vi "WheelShooter Shoot.vi"(1 "cluster in":T9, 2 "Range":dbl) -> (0 "error out":errorcluster)   [LabVIEW 2015]
doc: "Spins up the firing motors and then shoots over one second."
uses:
  <vilib>/Rock Robotics/WPI/MotorControl/WPI_MotorControlDeviceRef.ctl
  <vilib>/Rock Robotics/WPI/MotorControl/WPI_MotorControlType.ctl
  <vilib>/Rock Robotics/SystemInterfaces/DIO/FPGA_DIOPWMChannel.ctl
  <vilib>/Rock Robotics/WPI/PWM/WPI_PWMDeadband.ctl
  <vilib>/Rock Robotics/WPI/CAN/Jaguar/SubVIs/WPI_CANJaguar_ControlMode.ctl
  <vilib>/Rock Robotics/WPI/CAN/TalonSRX/WPI_CANTalonSRX_APIControlMode.ctl
  <vilib>/Rock Robotics/WPI/PWM/Servo/WPI_ServoDeviceRef.ctl
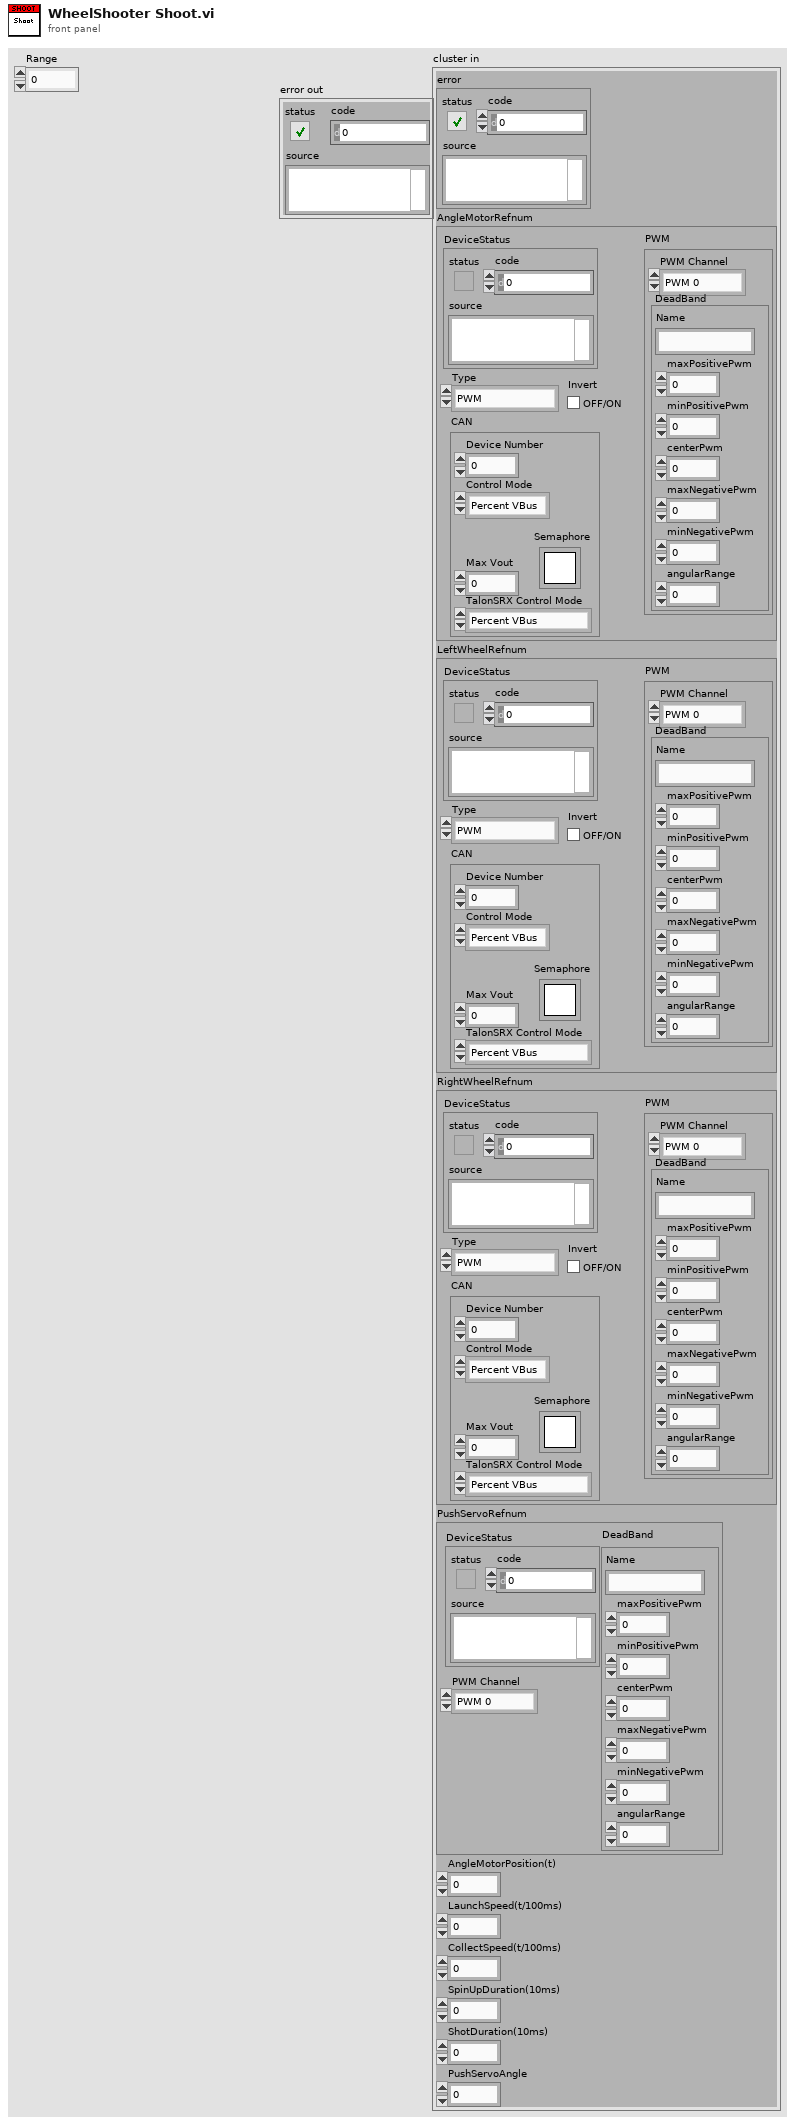
[diagram p1: front panel]
types:
  T1 = typedef "WPI_MotorControlDeviceRef.ctl" = cluster{"DeviceStatus":errorcluster, "Type":T2, "PWM":cluster{"PWM Channel":T3, "DeadBand":T4}, "CAN":cluster{"Device Number":u8, "Control Mode":T5, "Semaphore":T6, "Max Vout":dbl, "TalonSRX Control Mode":T7}, "Invert":bool}
  T2 = typedef "WPI_MotorControlType.ctl" = enum16{"PWM", "CAN", "CANTalonSRX"}
  T3 = typedef "FPGA_DIOPWMChannel.ctl" = enum8{"PWM 0", "PWM 1", "PWM 2", "PWM 3", "PWM 4", "PWM 5", "PWM 6", "PWM 7", "PWM 8", "PWM 9", "PWM MXP 0", "PWM MXP 1", "PWM MXP 2", "PWM MXP 3", "PWM MXP 4", "PWM MXP 5", "PWM MXP 6", "PWM MXP 7", "PWM MXP 8", "PWM MXP 9", "Invalid"}
  T4 = typedef "WPI_PWMDeadband.ctl" = cluster{"Name":string, "maxPositivePwm":i32, "minPositivePwm":i32, "centerPwm":i32, "maxNegativePwm":i32, "minNegativePwm":i32, "angularRange":u16}
  T5 = typedef "WPI_CANJaguar_ControlMode.ctl" = enum8{"Percent VBus", "Current", "Speed", "Position", "Voltage"}
  T6 = typedef "Semaphore RefNum" = refnum<k1>
  T7 = typedef "WPI_CANTalonSRX_APIControlMode.ctl" = enum8{"Percent VBus", "Speed", "Position", "Slave", "Unchanged / Invalid", "Voltage Compensation", "Current", "Motion Profile"}
  T8 = typedef "WPI_ServoDeviceRef.ctl" = cluster{"DeviceStatus":errorcluster, "PWM Channel":T3, "DeadBand":T4}
  T9 = cluster{"error":errorcluster, "AngleMotorRefnum":T1, "LeftWheelRefnum":T1, "RightWheelRefnum":T1, "PushServoRefnum":T8, "AngleMotorPosition(t)":dbl, "LaunchSpeed(t/100ms)":dbl, "CollectSpeed(t/100ms)":dbl, "SpinUpDuration(10ms)":i32, "ShotDuration(10ms)":i32, "PushServoAngle":i32}
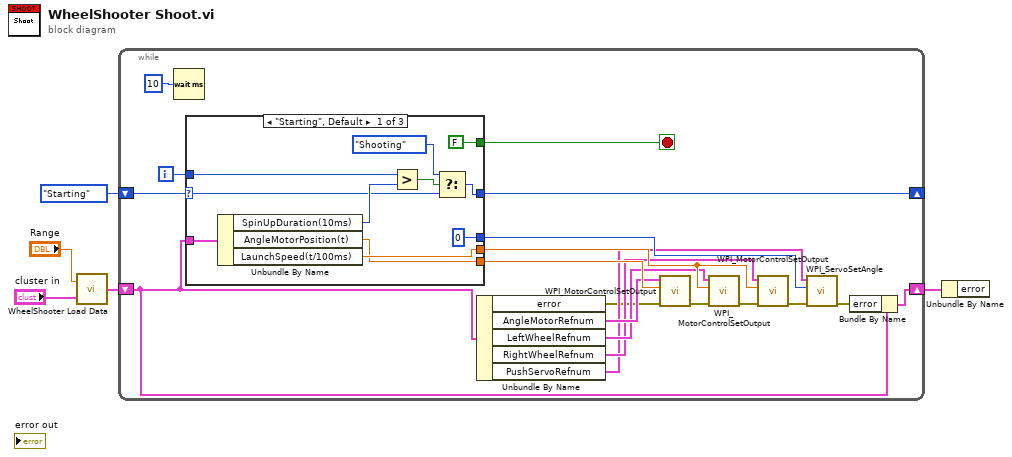
[diagram p0: block diagram]
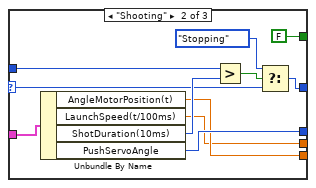
[diagram p2: hidden frame]
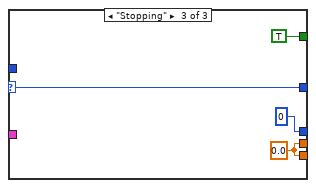
[diagram p3: hidden frame]
diagram:
  n1 = call "WheelShooter Load Data.vi"("cluster in"="cluster in", "Range"="Range") -> ("cluster out"=w3:T9)
  n2 = while {
    shift-right: [w20] -> _
    shift-left: enum16{"Starting", "Shooting", "Stopping"}."Starting" -> [w24]
    shift-right: [w13] -> w2
    shift-left: w3 -> [w12]
    i -> [w21]
    stop <- w6 stop-if-true
    n3 = Wait (ms)(milliseconds to wait=u32 10) -> ()  [unwired: 1 out]
    n4 = case shown="\"Starting\", Default" w24 {
      selector: w24 -> [w31 w43 w49]
      tunnel: [0 ("Angle") w40 0 ("Angle")] -> w23
      tunnel: w21 -> [w35 w44 _]
      tunnel: w12 -> [w33 w46 _]
      tunnel: [w29 w42 w49] -> w20
      tunnel: [w28 w37 w48] -> w19
      tunnel: [w27 w38 w48] -> w18
      tunnel: [FALSE FALSE TRUE] -> w6
      frame "Starting", Default {
        n5 = Unbundle By Name(w33) -> ("SpinUpDuration(10ms)"=w32:i32, "AngleMotorPosition(t)"=w27:dbl, "LaunchSpeed(t/100ms)"=w28:dbl)
        n6 = Greater?(x=w35, y=w32) -> (0:w30:bool)
        n7 = Select(t=enum16{"Starting", "Shooting", "Stopping"}."Shooting", s=w30, f=w31) -> (s? t:f=w29:enum16{"Starting", "Shooting", "Stopping"})
      }
      frame "Shooting" {
        n8 = Unbundle By Name(w46) -> ("AngleMotorPosition(t)"=w38:dbl, "LaunchSpeed(t/100ms)"=w37:dbl, "ShotDuration(10ms)"=w45:i32, "PushServoAngle"=w40:i32)
        n9 = Greater?(x=w44, y=w45) -> (0:w39:bool)
        n10 = Select(t=enum16{"Starting", "Shooting", "Stopping"}."Stopping", s=w39, f=w43) -> (s? t:f=w42:enum16{"Starting", "Shooting", "Stopping"})
      }
      frame "Stopping" {
        w48 = 0.0 ("AngleMotorT")
      }
    }
    n11 = Unbundle By Name(w12) -> ("error"=w7:errorcluster, "AngleMotorRefnum"=w17:T1, "LeftWheelRefnum"=w16:T1, "RightWheelRefnum"=w15:T1, "PushServoRefnum"=w14:T8)
    n12 = call <vilib>:"WPI_MotorControlSetOutput.vi"("error in (no error)"=w7, "Output"=w18, "MotorControlDevRef"=w17) -> ("error out"=w8:errorcluster)  [unwired: 6 in, 2 out]
    n13 = call <vilib>:"WPI_MotorControlSetOutput.vi"("error in (no error)"=w8, "Output"=w19, "MotorControlDevRef"=w16) -> ("error out"=w9:errorcluster)  [unwired: 6 in, 2 out]
    n14 = call <vilib>:"WPI_MotorControlSetOutput.vi"("error in (no error)"=w9, "Output"=w19, "MotorControlDevRef"=w15) -> ("error out"=w10:errorcluster)  [unwired: 6 in, 2 out]
    n15 = call <vilib>:"WPI_ServoSetAngle.vi"("error in (no error)"=w10, "Angle"=w23, "ServoDeviceRef"=w14) -> ("error out"=w11:errorcluster)  [unwired: 7 in, 1 out]
    n16 = Bundle By Name(cluster=w12, "error"=w11) -> (w13:T9)
  }
  n17 = Unbundle By Name(w2) -> ()  [unwired: 1 out]
